vi "IVA_Actividad_02.vi"() -> ()   [LabVIEW 2025]
panel:
  in  "DL1":bool
  in  "DL2":bool
  in  "SP2":bool
  out "f":dbl
  out "M":bool
  out "V2":bool
  out "V1":bool
  out "VB":bool
  out "VA":bool
  in  "Enum":T1(ring)
  in  "stop":bool
  in  "SP1":bool
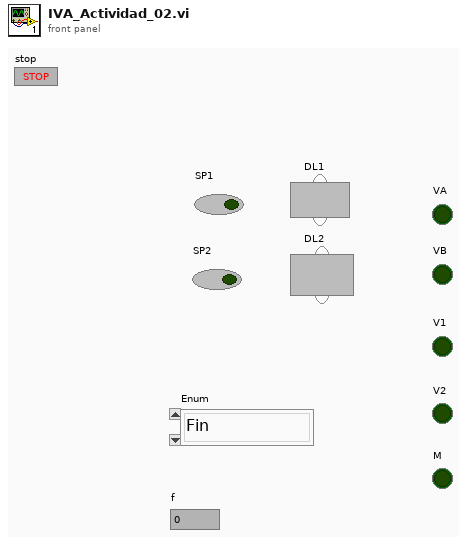
[diagram p1: front panel]
types:
  T1 = enum16{"Fin", "Motor", "V1_Abierto", "VB_abierto", "VA_Abierto", "Reposo", "V2_abierto"}
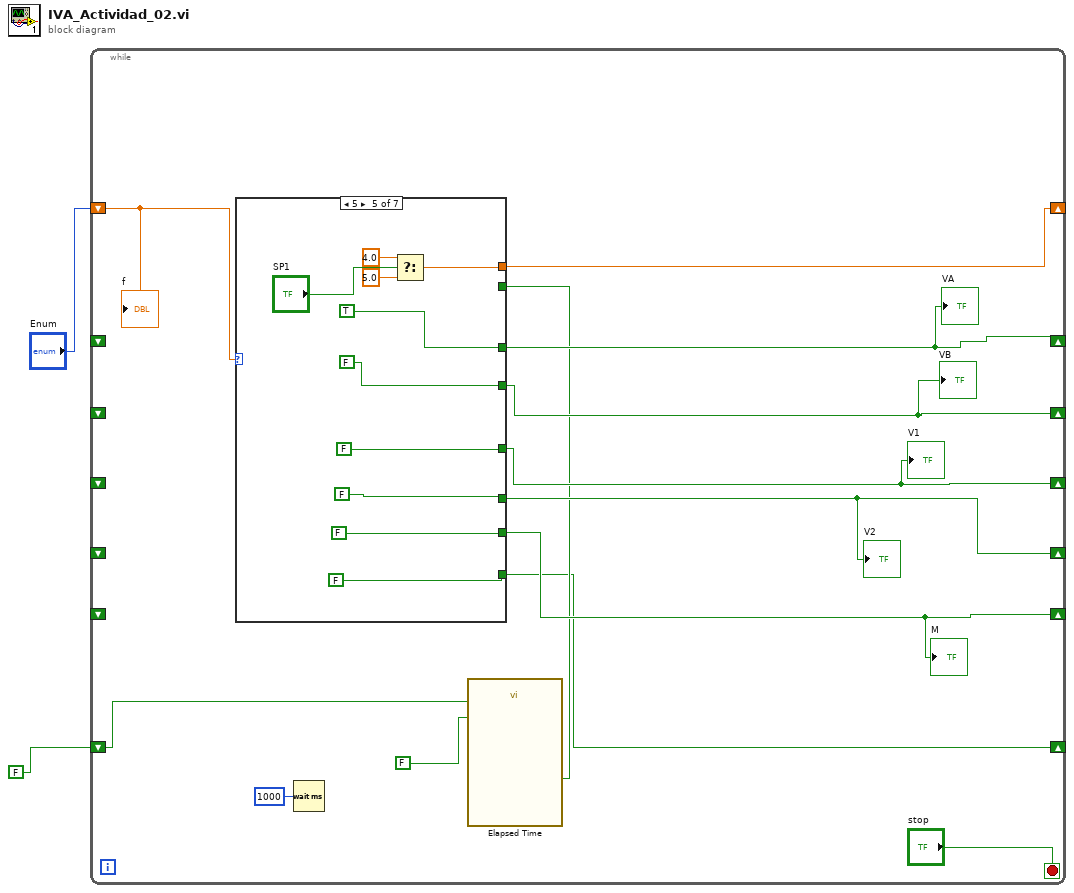
[diagram p0: block diagram]
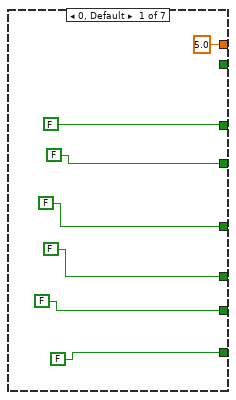
[diagram p2: hidden frame]
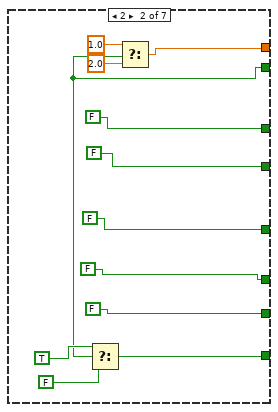
[diagram p3: hidden frame]
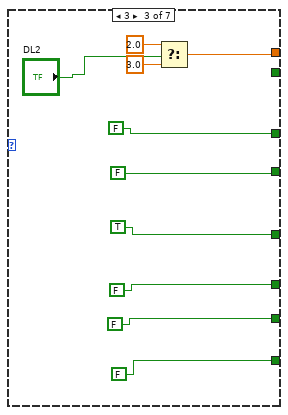
[diagram p4: hidden frame]
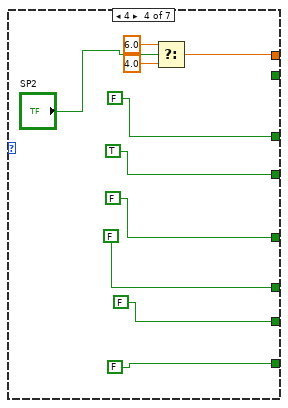
[diagram p5: hidden frame]
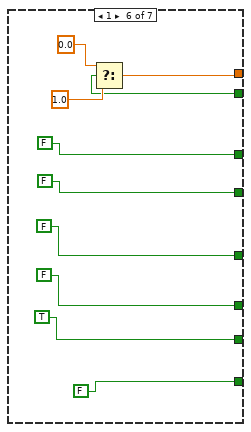
[diagram p6: hidden frame]
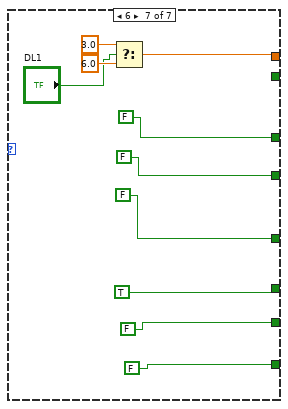
[diagram p7: hidden frame]
diagram:
  n1 = while {
    shift-right: [w8] -> _
    shift-left: "Enum" -> [w15]
    shift-right: [w14] -> _
    shift-left: _ -> [_]
    shift-right: [w13] -> _
    shift-left: _ -> [_]
    shift-right: [w11] -> _
    shift-left: _ -> [_]
    shift-right: [w10] -> _
    shift-left: _ -> [_]
    shift-right: [w9] -> _
    shift-left: _ -> [_]
    shift-right: [w4] -> _
    shift-left: FALSE -> [w7]
    stop <- "stop" stop-if-true
    n2 = Wait (ms)(milliseconds to wait=u32 1000) -> ()  [unwired: 1 out]
    n3 = call "Elapsed Time"("Reset"=w7, "Auto Reset"=FALSE) -> ("Time has Elapsed"=w5:bool)  [unwired: 10 in, 7 out]
    n4 = case shown="5" w15 {
      tunnel: [FALSE FALSE FALSE FALSE TRUE FALSE FALSE] -> w14
      tunnel: [FALSE FALSE FALSE TRUE FALSE FALSE FALSE] -> w13
      tunnel: [FALSE FALSE TRUE FALSE FALSE FALSE FALSE] -> w11
      tunnel: [FALSE FALSE FALSE FALSE FALSE FALSE TRUE] -> w10
      tunnel: [FALSE FALSE FALSE FALSE FALSE TRUE FALSE] -> w9
      tunnel: [5.0 ("f") w29 w39 w47 w58 w67 w80] -> w8
      tunnel: w5 -> [_ w23 _ _ _ w66 _]
      tunnel: [FALSE w24 FALSE FALSE FALSE FALSE FALSE] -> w4
      frame 0, Default {
      }
      frame 2 {
        n5 = Select(t=TRUE, s=w23, f=FALSE) -> (s? t:f=w24:bool)
        n6 = Select(t=1.0, s=w23, f=2.0) -> (s? t:f=w29:dbl)
      }
      frame 3 {
        n7 = Select(t=2.0, s="DL2", f=3.0) -> (s? t:f=w39:dbl)
      }
      frame 4 {
        n8 = Select(t=6.0, s="SP2", f=4.0) -> (s? t:f=w47:dbl)
      }
      frame 5 {
        n9 = Select(t=4.0, s="SP1", f=5.0) -> (s? t:f=w58:dbl)
      }
      frame 1 {
        n10 = Select(t=0.0, s=w66, f=1.0) -> (s? t:f=w67:dbl)
      }
      frame 6 {
        n11 = Select(t=3.0, s="DL1", f=6.0) -> (s? t:f=w80:dbl)
      }
    }
    "VB" <- w13
    "V1" <- w11
    "V2" <- w10
    "M" <- w9
    "VA" <- w14
    "f" <- w15
  }
